vi "Back Transform Eigenvectors.vi"   [LabVIEW 2018, in "NI_AALPro.lvlib"]
doc: "Transforms the eigenvectors of a balanced matrix to those of the original matrix. Wire data to the <B>Eigenvectors</B> input to determine the polymorphic instance to use or manually select the instance."
uses:
  NI_AALPro.lvlib
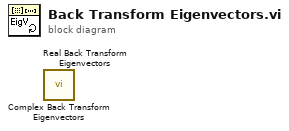
[diagram p0: block diagram]
diagram:
  n1 = call "Complex Back Transform Eigenvectors.vi"() -> ()  [unwired: 10 in, 2 out]
  n2 = call "Real Back Transform Eigenvectors.vi"() -> ()  [unwired: 10 in, 2 out]
